vi "Handle.vi"(8 "error in (no error)":errorcluster, 10 "Zero Timeout Message Handler in":refnum<class "Zero Timeout Message Handler.lvclass">, 11 "Message in":refnum<class "Set Timeout Message Msg.lvclass">) -> (0 "error out":errorcluster, 2 "Zero Timeout Message Handler out":refnum<class "Zero Timeout Message Handler.lvclass">)   [LabVIEW 2024, in "Zero Timeout Message Handler.lvlib" / "Set Timeout Message Msg.lvclass"]
uses:
  Zero Timeout Message Handler/Zero Timeout Message Handler.lvclass
  Set Timeout Message Msg.lvclass
  Set Timeout Message Msg.lvclass/Set Timeout Message Msg.ctl
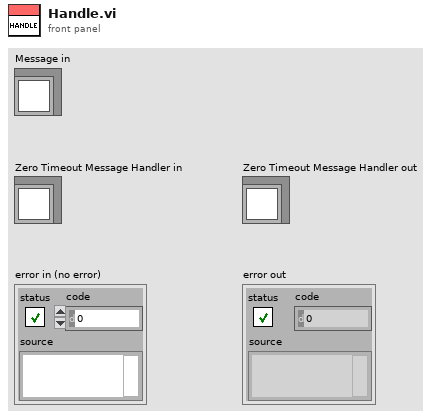
[diagram p1: front panel]
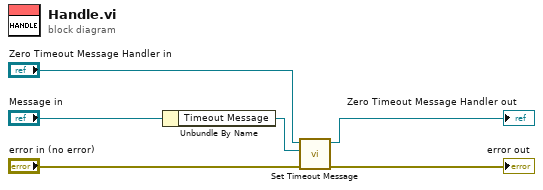
[diagram p0: block diagram]
diagram:
  n1 = Unbundle By Name("Message in") -> ("Timeout Message"=w1:refnum<class "~Message.lvclass">)
  n2 = call-dynamic "Set Timeout Message.vi"("error in (no error)"="error in (no error)", "Timeout Message"=w1, "Zero Timeout Message Handler in"="Zero Timeout Message Handler in") -> ("error out"=→"error out":errorcluster, "Zero Timeout Message Handler out"=→"Zero Timeout Message Handler out":refnum<class "Zero Timeout Message Handler.lvclass">)  [unwired: 7 in]
